vi "CameraKill.vi"(8 "error in (no error)":errorcluster, 11 "IMAQdx in":refnum<class "IMAQdx.lvclass">) -> (0 "error out":errorcluster, 3 "IMAQdx out":refnum<class "IMAQdx.lvclass">)   [LabVIEW 2010, in "IMAQdx.lvclass"]
uses:
  <userlib>/bias/classes/IMAQdx/IMAQdx.lvclass
  <vilib>/userDefined/High Color/IMAQdx.ctl
  <userlib>/bias/classes/IMAQdx/IMAQdx.lvclass/IMAQdx.ctl
  <vilib>/vision/driver/NI_Vision_Acquisition_Software.lvlib
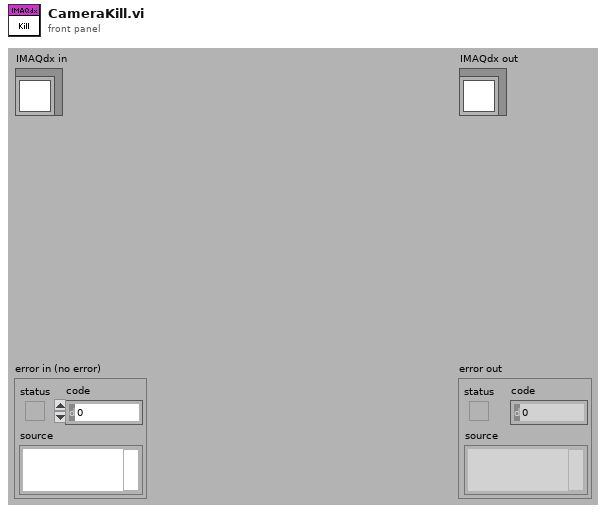
[diagram p1: front panel]
types:
  T1 = typedef "IMAQdx.ctl" = refnum<k21>
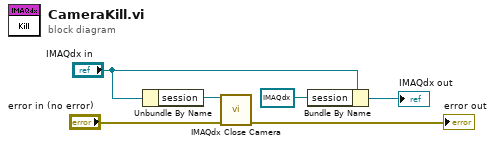
[diagram p0: block diagram]
diagram:
  n1 = Unbundle By Name("IMAQdx in") -> ("session"=w6:refnum<k21>)
  n2 = call <vilib>:"IMAQdx Close Camera.vi"("error in"="error in (no error)", "Session In"=w6) -> ("error out"=→"error out":errorcluster)  [unwired: 9 in]
  n3 = Bundle By Name(cluster="IMAQdx in", "session"=T1 refnum) -> (→"IMAQdx out":refnum<class "IMAQdx.lvclass">)
